vi "Get Pulse Length.vi"(7 "Ref Pulse Length":refnum<vi>, 8 "error in":errorcluster, 9 "Head Channel":i16, 10 "Pulsar Handle":i16, 11 "OphirFastX (in)":refnum<k7>) -> (0 "error out":errorcluster, 3 "OphirFastX (out)":refnum<k7>)   [LabVIEW 2009]
panel:
  # "Guillaume Plateau - yguig2@yahoo.fr"
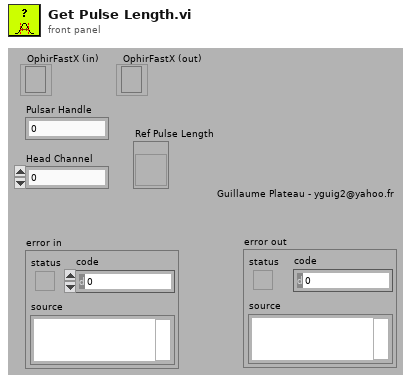
[diagram p1: front panel]
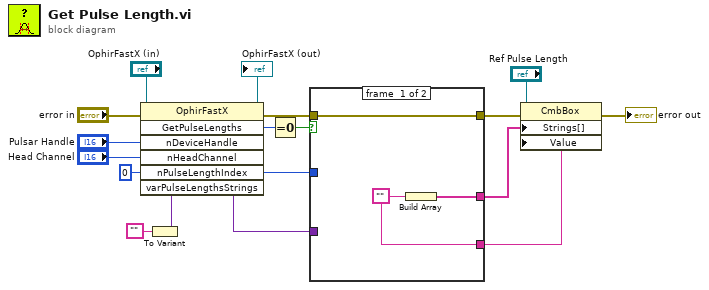
[diagram p0: block diagram]
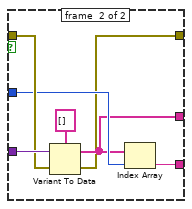
[diagram p2: hidden frame]
diagram:
  n1 = To Variant(anything="") -> (Variant=w11:variant)
  n2 = invoke class="OphirFastX" method="GetPulseLengths"(reference="OphirFastX (in)", error in="error in", "nDeviceHandle"="Pulsar Handle", "nHeadChannel"="Head Channel", "nPulseLengthIndex"=i16 0, "varPulseLengthsStrings"=w11) -> (reference out=→"OphirFastX (out)":refnum<k7>, error out=w14:errorcluster, "GetPulseLengths"=w12:i32, "nPulseLengthIndex"=w15:i16, "varPulseLengthsStrings"=w16:variant)  [unwired: 1 in, 2 out]
  n3 = Equal To 0?(x=w12) -> (x = 0?=w13:bool)
  n4 = case shown="True" w13 {
    tunnel: w16 -> [_ w28]
    tunnel: w14 -> [w19 w27]
    tunnel: w15 -> [_ w25]
    tunnel: [w21 w24] -> w1
    tunnel: [w20 w23] -> w4
    tunnel: [w19 w22] -> w6
    frame #0 {
      w20 = ""
      n5 = Build Array(w20) -> (w21:string[])
    }
    frame #1 {
      n6 = Variant To Data(error in=w27, Variant=w28, type=string[] []) -> (error out=w22:errorcluster, data=w24:string[])
      n7 = Index Array(array=w24, index=w25) -> (element=w23:string)
    }
  }
  n8 = property class="CmbBox"(reference="Ref Pulse Length", error in=w6, "Strings[]"=w1, "Value"=w4) -> (error out=→"error out":errorcluster)  [unwired: 1 out]
